vi "Stop Core.vi"(10 "final error code":i32, 11 "Test LNA in":refnum<class "TestLNA.lvclass">) -> (3 "Test LNA out":refnum<class "TestLNA.lvclass">)   [LabVIEW 2015, in "TestLNA.lvlib" / "TestLNA.lvclass"]
doc: "(<B>Filename</B>: Actor Framework.lvlib:Actor.lvclass:Stop Core.vi)\n\nDefines what the actor does before it stops. Use the <B>final error code</B> input to determine whether the actor shut down in response to an error.\n\nBy default, this method does nothing. A descendant class may override it to define behavior, such as shutting down any processes the actor initiated in its override of the Actor Core method."
uses:
  TestLNA.lvclass
  <vilib>/ActorFramework/Time-Delayed Send Message/Time-Delay Override Options.ctl
  TestLNA.lvclass/TestLNA.ctl
  CSPP_Core/Actors/CS++BaseActor/CS++BaseActor.lvclass
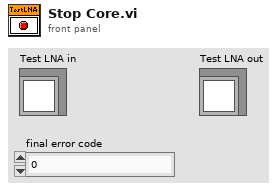
[diagram p1: front panel]
types:
  T1 = typedef "Time-Delay Override Options.ctl" = enum16{"Send next copy now", "Skip next scheduled copy", "Send next copy now and stop all further copies", "Stop all further copies"}
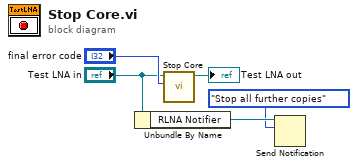
[diagram p0: block diagram]
diagram:
  n1 = Unbundle By Name("Test LNA in") -> ("RLNA Notifier"=w2:refnum<notifier>)
  n2 = call-parent "Stop Core.vi"("final error code"="final error code", "CS++BaseActor in"="Test LNA in") -> ("CS++BaseActor out"=→"Test LNA out":refnum<class "TestLNA.lvclass">)  [unwired: 9 in]
  n3 = Send Notification(notification=Time-Delay_Override_Options."Stop all further copies", notifier=w2) -> ()  [unwired: 1 in, 2 out]
